vi "SyncLoopHandler.vi"(8 "error in (no error)":errorcluster, 10 "LoopProperties":refnum<class "SyncPluginBase.lvclass">, 11 "PXI_MultiTrig in":refnum<class "PXI_MultiTrig.lvclass">) -> (0 "error out":errorcluster, 3 "PXI_MultiTrig out":refnum<class "PXI_MultiTrig.lvclass">)   [LabVIEW 2014, in "SyncPlugins.lvlib" / "PXI_MultiTrig.lvclass"]
uses:
  PXI_MultiTrig.lvclass
  SyncPluginBase/SyncPluginBase.lvclass
  SyncPluginBase/SyncPluginBase.lvclass/SyncPluginBase.ctl
  PXI_MultiTrig.lvclass/PXI_MultiTrig.ctl
  Accessors/Read RefClkSession.vi
  Accessors/Read Clocks.vi
  SyncPluginBase/Accessors/Write Run.vi
  SyncPluginBase/Accessors/Write Monitor Loop.vi
  SyncPluginBase/Accessors/Write Locked.vi
  SyncPluginBase/Accessors/Read Locked.vi
  SyncPluginBase/Accessors/Read Run.vi
  SyncPluginBase/Accessors/Read LostLock.vi
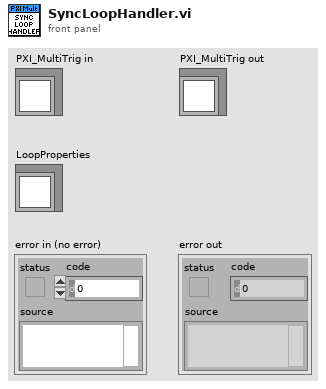
[diagram p1: front panel]
types:
  T1 = typedef "SyncPlugins.lvlib/PXI_MultiTrig.lvclass/clClocks.ctl" = cluster{"Name":string, "RefClk":string, "ClkTerminal":string, "Frequency":dbl, "DutyCycle":dbl, "ClkType":string, "Initiated":bool, "TrigTime":bool}
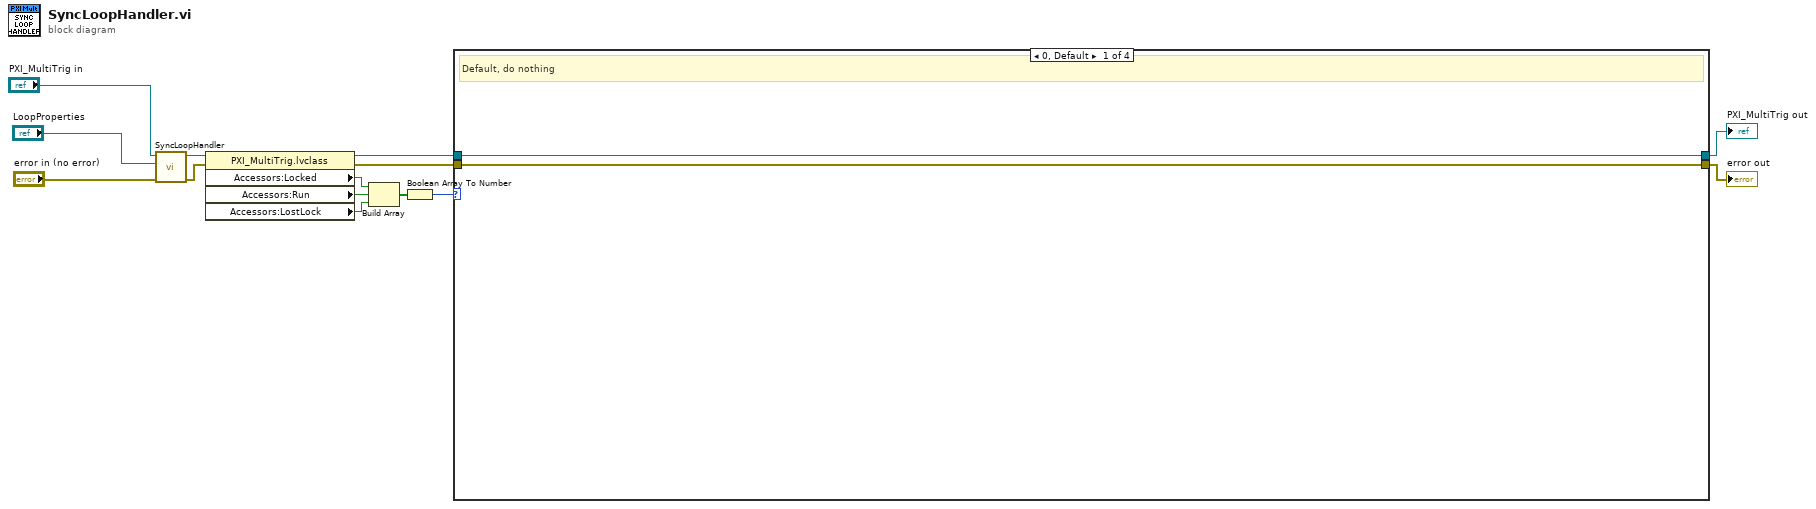
[diagram p0: block diagram]
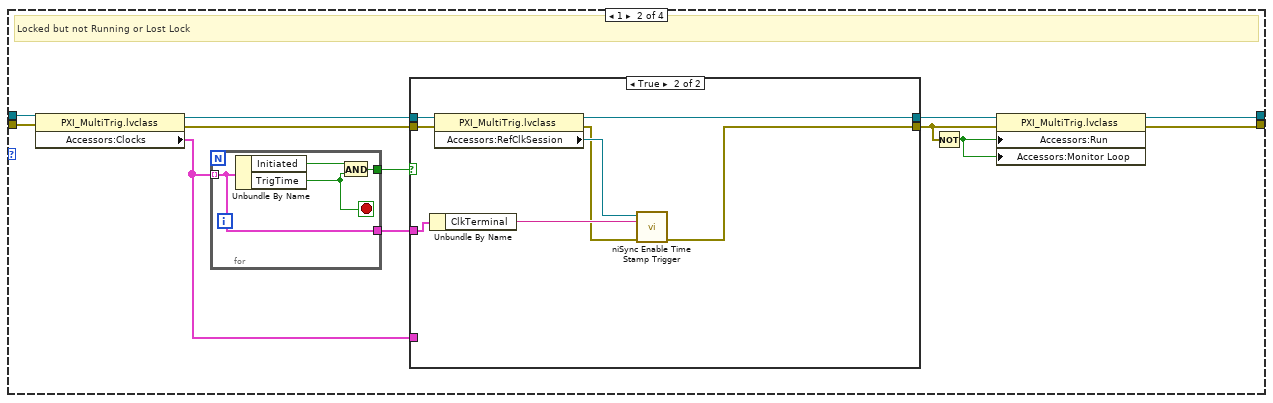
[diagram p2: hidden frame]
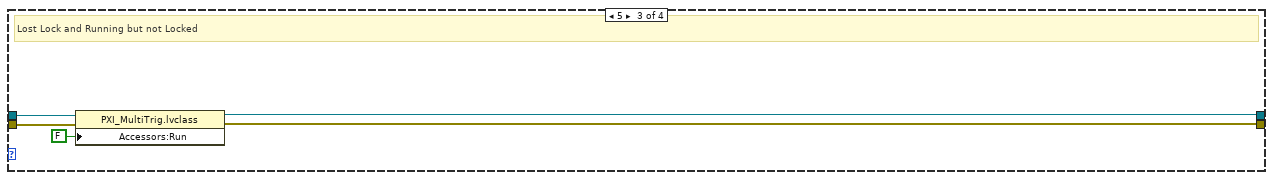
[diagram p4: hidden frame]
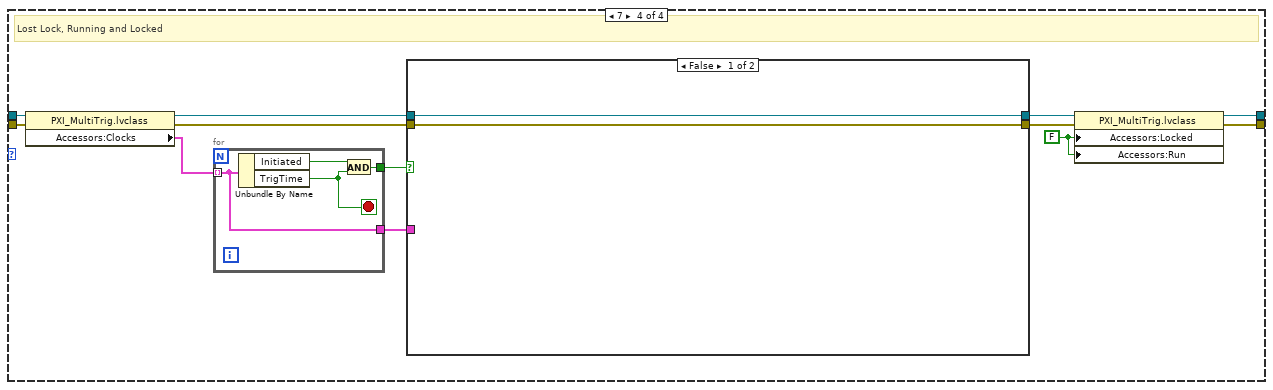
[diagram p5: hidden frame]
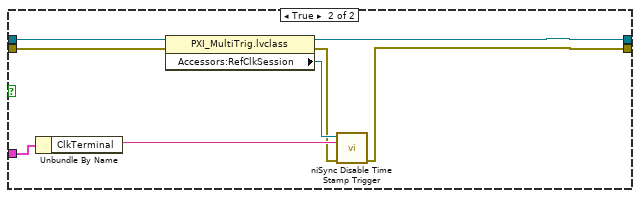
[diagram p6: hidden frame]
diagram:
  n1 = call-parent "SyncLoopHandler.vi"("error in (no error)"="error in (no error)", "LoopProperties"="LoopProperties", "SyncPluginBase in"="PXI_MultiTrig in") -> ("error out"=w11:errorcluster, "SyncPluginBase out"=w14:refnum<class "PXI_MultiTrig.lvclass">)  [unwired: 7 in]
  n2 = property class="PXI_MultiTrig.lvclass"(reference=w14, error in=w11) -> (reference out=w5:refnum<class "PXI_MultiTrig.lvclass">, error out=w4:errorcluster, "Accessors:Locked"=w10:bool, "Accessors:Run"=w8:bool, "Accessors:LostLock"=w9:bool)
  n3 = Build Array(w10, w8, w9) -> (w7:bool[])
  n4 = Boolean Array To Number(Boolean array=w7) -> (number=w6:u32)
  n5 = case shown="0, Default" w6 {
    tunnel: w5 -> [w16 w28 w47 w58]
    tunnel: w4 -> [w15 w22 w46 w59]
    tunnel: [w16 w20 w44 w49] -> w3
    tunnel: [w15 w19 w43 w48] -> w2
    frame 0, Default {
      # "Default, do nothing"
    }
    frame 1 {
      # "Locked but not Running or Lost Lock"
      n6 = property class="PXI_MultiTrig.lvclass"(reference=w28, error in=w22) -> (reference out=w26:refnum<class "PXI_MultiTrig.lvclass">, error out=w25:errorcluster, "Accessors:Clocks"=w24:T1[])
      n7 = for {
        tunnel: w24 -> [w42] mode=indexing
        tunnel: [w42] -> w23
        tunnel: [w40] -> w27
        stop <- w39 stop-if-true
        n8 = Unbundle By Name(w42) -> ("Initiated"=w41:bool, "TrigTime"=w39:bool)
        n9 = And(x=w41, y=w39) -> (x .and. y?=w40:bool)
      }
      n10 = case shown="True" w27 {
        tunnel: w23 -> [_ w35]
        tunnel: w26 -> [w30 w38]
        tunnel: w25 -> [w29 w36]
        tunnel: [w29 w31] -> w18
        tunnel: [w30 w32] -> w21
        tunnel: w24 -> [_ _]
        frame False {
        }
        frame True {
          n11 = Unbundle By Name(w35) -> ("ClkTerminal"=w37:string)
          n12 = property class="PXI_MultiTrig.lvclass"(reference=w38, error in=w36) -> (reference out=w32:refnum<class "PXI_MultiTrig.lvclass">, error out=w33:errorcluster, "Accessors:RefClkSession"=w34:refnum<k15>)
          n13 = call <instrlib>:"niSync Enable Time Stamp Trigger.vi"("error in (no error)"=w33, "terminal"=w37, "instrument handle"=w34) -> ("error out"=w31:errorcluster)  [unwired: 6 in, 1 out]
        }
      }
      n14 = Not(x=w18) -> (.not. x?=w17:bool)
      n15 = property class="PXI_MultiTrig.lvclass"(reference=w21, error in=w18, "Accessors:Run"=w17, "Accessors:Monitor Loop"=w17) -> (reference out=w20:refnum<class "PXI_MultiTrig.lvclass">, error out=w19:errorcluster)
    }
    frame 5 {
      # "Lost Lock and Running but not Locked"
      n16 = property class="PXI_MultiTrig.lvclass"(reference=w47, error in=w46, "Accessors:Run"=FALSE ("Run")) -> (reference out=w44:refnum<class "PXI_MultiTrig.lvclass">, error out=w43:errorcluster)
    }
    frame 7 {
      w50 = FALSE
      # "Lost Lock, Running and Locked"
      n17 = property class="PXI_MultiTrig.lvclass"(reference=w58, error in=w59) -> (reference out=w57:refnum<class "PXI_MultiTrig.lvclass">, error out=w56:errorcluster, "Accessors:Clocks"=w53:T1[])
      n18 = for {
        tunnel: w53 -> [w73] mode=indexing
        tunnel: [w73] -> w54
        tunnel: [w71] -> w55
        stop <- w70 stop-if-true
        n19 = Unbundle By Name(w73) -> ("Initiated"=w72:bool, "TrigTime"=w70:bool)
        n20 = And(x=w72, y=w70) -> (x .and. y?=w71:bool)
      }
      n21 = case shown="False" w55 {
        tunnel: w54 -> [_ w66]
        tunnel: w57 -> [w61 w69]
        tunnel: w56 -> [w60 w67]
        tunnel: [w60 w62] -> w51
        tunnel: [w61 w63] -> w52
        frame False {
        }
        frame True {
          n22 = Unbundle By Name(w66) -> ("ClkTerminal"=w68:string)
          n23 = property class="PXI_MultiTrig.lvclass"(reference=w69, error in=w67) -> (reference out=w63:refnum<class "PXI_MultiTrig.lvclass">, error out=w64:errorcluster, "Accessors:RefClkSession"=w65:refnum<k15>)
          n24 = call <instrlib>:"niSync Disable Time Stamp Trigger.vi"("error in (no error)"=w64, "terminal"=w68, "instrument handle"=w65) -> ("error out"=w62:errorcluster)  [unwired: 6 in, 1 out]
        }
      }
      n25 = property class="PXI_MultiTrig.lvclass"(reference=w52, error in=w51, "Accessors:Locked"=w50, "Accessors:Run"=w50) -> (reference out=w49:refnum<class "PXI_MultiTrig.lvclass">, error out=w48:errorcluster)
    }
  }
  "error out" <- w2
  "PXI_MultiTrig out" <- w3
